vi "TreeSelectMoves.vi"(8 "error in (no error)":errorcluster, 10 "Gameboard":T1, 11 "Map":T2) -> (0 "error out":errorcluster, 2 "How rotated?":i8[](array[numeric]), 3 "Moves":i8[](array[numeric]))   [LabVIEW 2020]
uses:
  controls/DecisionTree.ctl
  controls/Gameboard Data.ctl
  controls/DecisionTreeRecord.ctl
  controls/Player.ctl
  GetEquivalentKeysNumeric.vi
  MakeSquare.vi
  Flatten2DArray.vi
  <vilib>/Utility/error.llb/Error Cluster From Error Code.vi
  GetAllIsometriesOf2DArray.vi
  <vilib>/ErrorRing/Error Ring.xnode
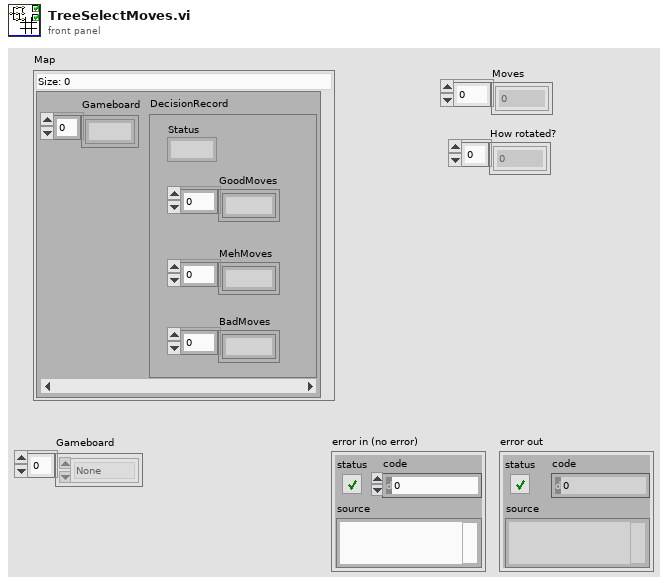
[diagram p1: front panel]
types:
  T1 = typedef "Gameboard Data.ctl" = enum16{"None", "Player 1", "Player 2"}[]
  T2 = typedef "DecisionTree.ctl" = map{T1, T3}
  T3 = typedef "DecisionTreeRecord.ctl" = cluster{"Status":T4, "GoodMoves":i8[], "MehMoves":i8[], "BadMoves":i8[]}
  T4 = typedef "Player.ctl" = enum16{"None", "Player 1", "Player 2"}
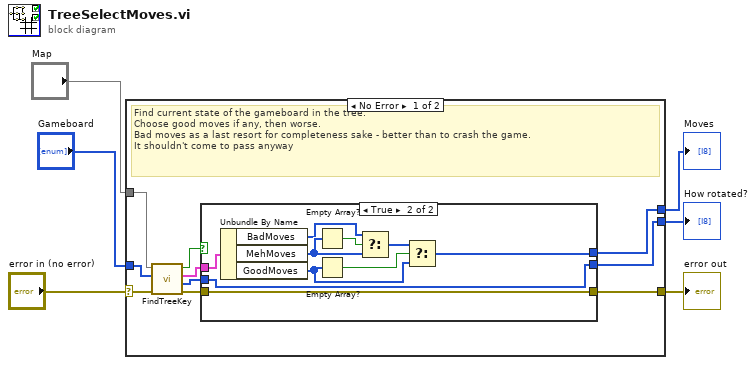
[diagram p0: block diagram]
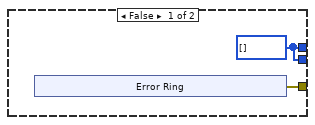
[diagram p2: hidden frame]
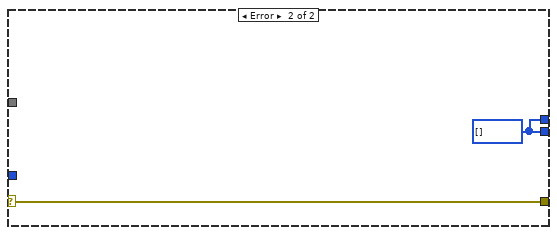
[diagram p3: hidden frame]
diagram:
  n1 = case shown="No Error" "error in (no error)" {
    selector: "error in (no error)" -> [w16 w35]
    tunnel: [w11 w35] -> w5
    tunnel: "Gameboard" -> [w15 _]
    tunnel: "Map" -> [w14 _]
    tunnel: [w10 w34] -> w2
    tunnel: [w7 w34] -> w1
    frame No Error {
      # "Find current state of the gameboard in the tree.\nChoose good moves if any, then worse.\nBad moves as a last resort for completeness sake - better than to crash the game.\nIt shouldn't come to pass anyway"
      n2 = call "FindTreeKey.vi"("error in (no error)"=w16, "Key"=w15, "Map"=w14) -> ("error out"=w12:errorcluster, "How rotated?"=w8:i8[], "DecisionRecord"=w9:T3, "IsFound?"=w13:bool)  [unwired: 5 in]
      n3 = case shown="True" w13 {
        tunnel: w12 -> [_ w33]
        tunnel: [w18 w33] -> w11
        tunnel: [w17 w27] -> w10
        tunnel: w9 -> [_ w32]
        tunnel: w8 -> [_ w24]
        tunnel: [w17 w24] -> w7
        frame False {
          w17 = i8[] [] ("Moves")
          n4 = xnode "Error Ring"() -> ("error out"=w18:errorcluster)
        }
        frame True {
          n5 = Unbundle By Name(w32) -> ("BadMoves"=w25:i8[], "MehMoves"=w26:i8[], "GoodMoves"=w30:i8[])
          n6 = Empty Array?(array=w26) -> (empty?=w28:bool)
          n7 = Empty Array?(array=w30) -> (empty?=w31:bool)
          n8 = Select(t=w25, s=w28, f=w26) -> (s? t:f=w29:i8[])
          n9 = Select(t=w29, s=w31, f=w30) -> (s? t:f=w27:i8[])
        }
      }
    }
    frame Error {
      w34 = i8[] [] ("GoodMoves")
    }
  }
  "error out" <- w5
  "Moves" <- w2
  "How rotated?" <- w1
